vi "SW_Clear_Specific_Errors.vi"(3 "Error In":errorcluster, 5 "Code section":enum16{"Not Specified", "HW Init"}(ring)) -> (0 "Error Out":errorcluster, 2 "specific error cleared?":bool)   [LabVIEW 2018, in "Tracker.lvlib"]
uses:
  Tracker.lvlib
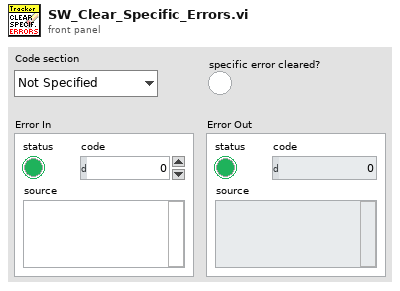
[diagram p1: front panel]
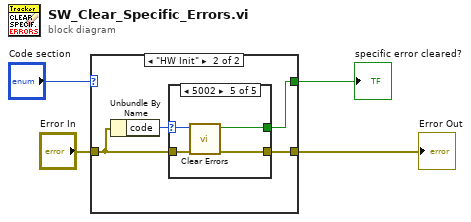
[diagram p0: block diagram]
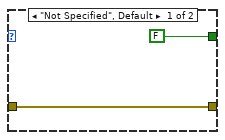
[diagram p2: hidden frame]
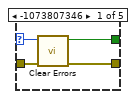
[diagram p3: hidden frame]
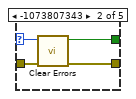
[diagram p4: hidden frame]
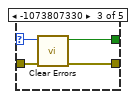
[diagram p5: hidden frame]
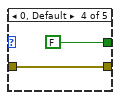
[diagram p6: hidden frame]
diagram:
  n1 = case shown="\"HW Init\"" "Code section" {
    tunnel: "Error In" -> [w6 w8]
    tunnel: [w6 w9] -> w1
    tunnel: [FALSE ("specific error cleared?") w7] -> w2
    frame "Not Specified", Default {
    }
    frame "HW Init" {
      n2 = Unbundle By Name(w8) -> ("code"=w10:i32)
      n3 = case shown="5002" w10 {
        selector: w10 -> [w12 w16 w20 _ w26]
        tunnel: [w13 w17 w21 w24 w27] -> w9
        tunnel: w8 -> [w14 w18 w22 w24 w28]
        tunnel: [w11 w15 w19 FALSE ("specific error cleared?") w25] -> w7
        frame -1073807346 {
          n4 = call <vilib>:"Clear Errors.vi"("error in (no error)"=w14, "specific error code to clear (0: all)"=w12) -> ("error out"=w13:errorcluster, "specific error cleared?"=w11:bool)  [unwired: 4 in]
        }
        frame -1073807343 {
          n5 = call <vilib>:"Clear Errors.vi"("error in (no error)"=w18, "specific error code to clear (0: all)"=w16) -> ("error out"=w17:errorcluster, "specific error cleared?"=w15:bool)  [unwired: 4 in]
        }
        frame -1073807330 {
          n6 = call <vilib>:"Clear Errors.vi"("error in (no error)"=w22, "specific error code to clear (0: all)"=w20) -> ("error out"=w21:errorcluster, "specific error cleared?"=w19:bool)  [unwired: 4 in]
        }
        frame 0, Default {
        }
        frame 5002 {
          n7 = call <vilib>:"Clear Errors.vi"("error in (no error)"=w28, "specific error code to clear (0: all)"=w26) -> ("error out"=w27:errorcluster, "specific error cleared?"=w25:bool)  [unwired: 4 in]
        }
      }
    }
  }
  "Error Out" <- w1
  "specific error cleared?" <- w2
